vi "Rpt _Get _CMBPCBAInfo.vi"(6 "DateTo":string, 7 "DateFrom":string, 8 "error in (no error)":errorcluster caption="错误输入（无错误）", 9 "Model":string, 10 "PO":string, 11 "Traceability 引用句柄":refnum<k24>) -> (0 "error out":errorcluster caption="错误输出", 2 ".NET:System.Data.DataSet":T1={"CaseSensitive"=FALSE, "Container"=refnum, "DataSetName"="", "DefaultViewManager"=refnum, "DesignMode"=FALSE, "EnforceConstraints"=FALSE, "ExtendedProperties"=refnum, "HasErrors"=FALSE, "IsInitialized"=FALSE, "Locale"=refnum, "Namespace"="", "Prefix"="", "Relations"=refnum, "RemotingFormat"=0, "SchemaSerializationMode"=1, "Site"=refnum, "Tables"=refnum} {"SchemaSerializationMode" items=["IncludeSchema"=1, "ExcludeSchema"=2]; "RemotingFormat" items=["Xml", "Binary"]}, 3 "Traceability 引用句柄输出":refnum<k24>)   [LabVIEW 2014, in "Traceability.lvlib"]
uses:
  D:/webservice/Traceability.dll
  Traceability.dll
  System.Data
  Traceability.lvlib
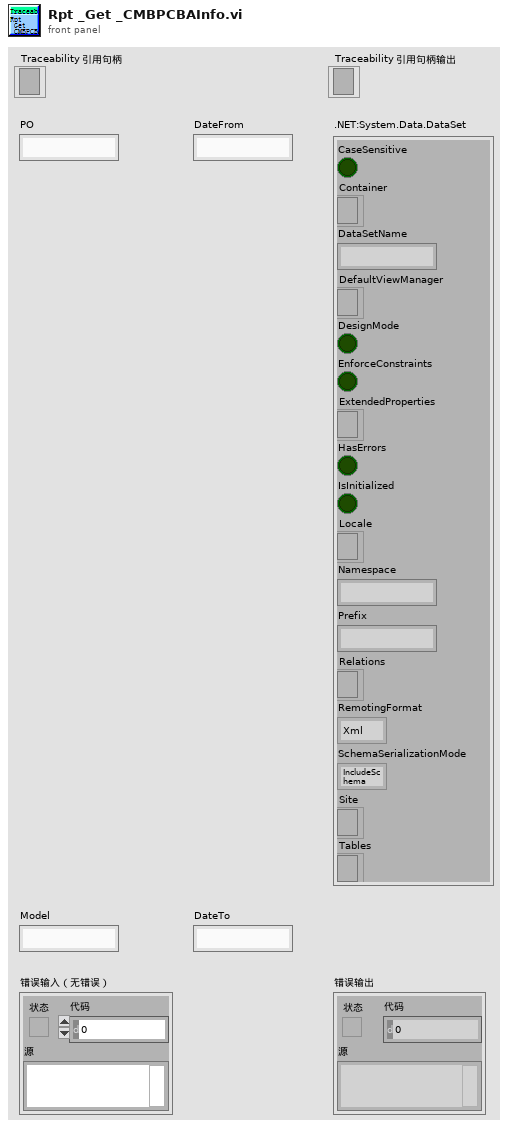
[diagram p1: front panel]
types:
  T1 = cluster{"CaseSensitive":bool, "Container":refnum<k24>, "DataSetName":string, "DefaultViewManager":refnum<k24>, "DesignMode":bool, "EnforceConstraints":bool, "ExtendedProperties":refnum<k24>, "HasErrors":bool, "IsInitialized":bool, "Locale":refnum<k24>, "Namespace":string, "Prefix":string, "Relations":refnum<k24>, "RemotingFormat":i32, "SchemaSerializationMode":i32, "Site":refnum<k24>, "Tables":refnum<k24>}
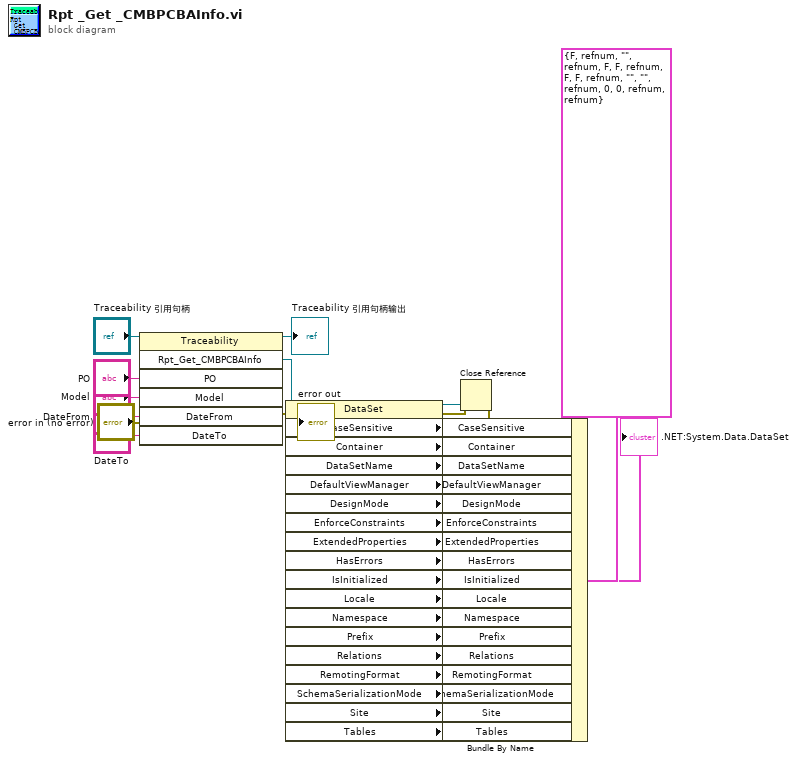
[diagram p0: block diagram]
diagram:
  n1 = invoke class="Traceability" method="Rpt_Get_CMBPCBAInfo"(reference="Traceability 引用句柄", error in="error in (no error)", "PO"="PO", "Model"="Model", "DateFrom"="DateFrom", "DateTo"="DateTo") -> (reference out=→"Traceability 引用句柄输出":refnum<k24>, error out=w4:errorcluster, "Rpt_Get_CMBPCBAInfo"=w28:refnum<k24>)  [unwired: 1 in, 4 out]
  n2 = property class="DataSet"(reference=w28, error in=w4) -> (reference out=w3:refnum<k24>, error out=w2:errorcluster, "CaseSensitive"=w25:bool, "Container"=w24:refnum<k24>, "DataSetName"=w23:string, "DefaultViewManager"=w22:refnum<k24>, "DesignMode"=w21:bool, "EnforceConstraints"=w20:bool, "ExtendedProperties"=w19:refnum<k24>, "HasErrors"=w18:bool, "IsInitialized"=w17:bool, "Locale"=w16:refnum<k24>, "Namespace"=w15:string, "Prefix"=w14:string, "Relations"=w13:refnum<k24>, "RemotingFormat"=w12:i32, "SchemaSerializationMode"=w11:i32, "Site"=w10:refnum<k24>, "Tables"=w9:refnum<k24>)
  n3 = Bundle By Name(cluster=T1 {"CaseSensitive"=FALSE, "Container"=refnum, "DataSetName"="", "DefaultViewManager"=refnum, "DesignMode"=FALSE, "EnforceConstraints"=FALSE, "ExtendedProperties"=refnum, "HasErrors"=FALSE, "IsInitialized"=FALSE, "Locale"=refnum, "Namespace"="", "Prefix"="", "Relations"=refnum, "RemotingFormat"=0, "SchemaSerializationMode"=0, "Site"=refnum, "Tables"=refnum} (".NET:System.Data.DataSet"), "CaseSensitive"=w25, "Container"=w24, "DataSetName"=w23, "DefaultViewManager"=w22, "DesignMode"=w21, "EnforceConstraints"=w20, "ExtendedProperties"=w19, "HasErrors"=w18, "IsInitialized"=w17, "Locale"=w16, "Namespace"=w15, "Prefix"=w14, "Relations"=w13, "RemotingFormat"=w12, "SchemaSerializationMode"=w11, "Site"=w10, "Tables"=w9) -> (→".NET:System.Data.DataSet":T1)
  n4 = Close Reference(reference=w3, error in (no error)=w2) -> (error out=→"error out":errorcluster)
